vi "test Scheduled Loopback with SDI.vi"(8 "error in":errorcluster, 11 "TestCase in":refnum<class "Single Board Loopback.lvclass">) -> (0 "error out":errorcluster, 3 "TestCase out":refnum<class "Single Board Loopback.lvclass">)   [LabVIEW 2020, in "Single Board Loopback.lvclass"]
uses:
  Single Board Loopback.lvclass
  C:/Users/nitest/Desktop/Git 2020/niveristand-custom-device-testing-tools/VeriStandTestCase/VeriStandTestCase.lvclass
  <vilib>/numeric/Random Number (Range) U64.vi
  <vilib>/numeric/sub_Random U32.vi
  <vilib>/addons/_JKI Toolkits/VI Tester/TestCase.llb/TestCase.lvclass
  niveristand-custom-device-testing-tools/VeriStandTestUtilities/VeriStandTestUtilities.lvlib
  C:/Program Files (x86)/National Instruments/LabVIEW 2020/vi.lib/addons/_JKI Toolkits/VI Tester/TestCase.llb/TestCase.lvclass
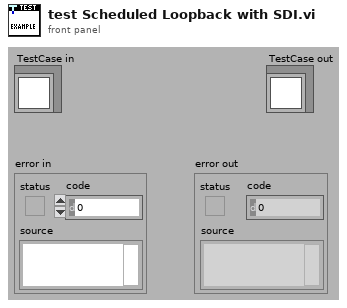
[diagram p1: front panel]
types:
  T1 = typedef "NI_VS Workspace ExecutionAPI.lvlib/WorkspaceAPI.ctl" = refnum<k24>
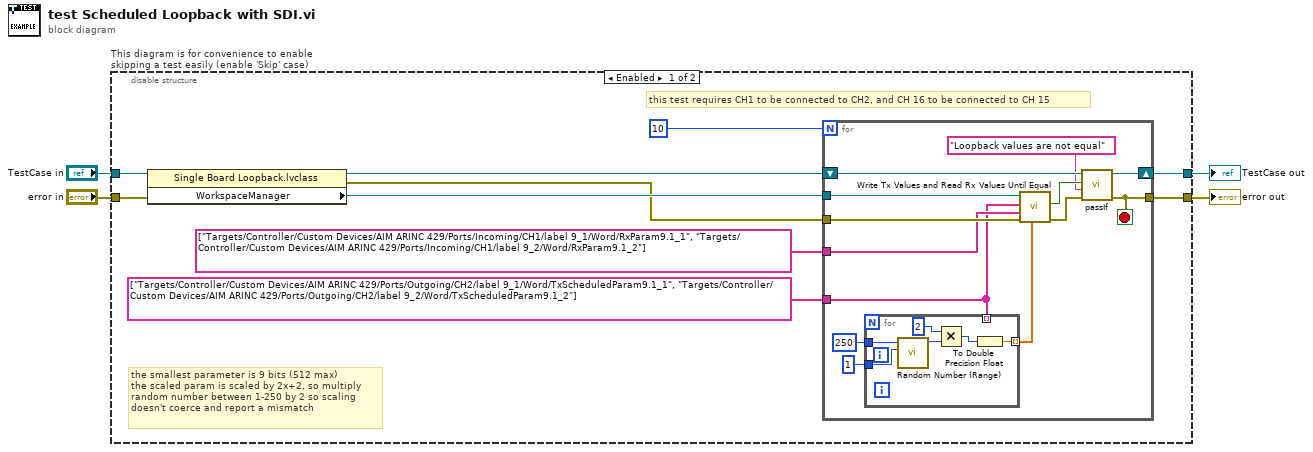
[diagram p0: block diagram]
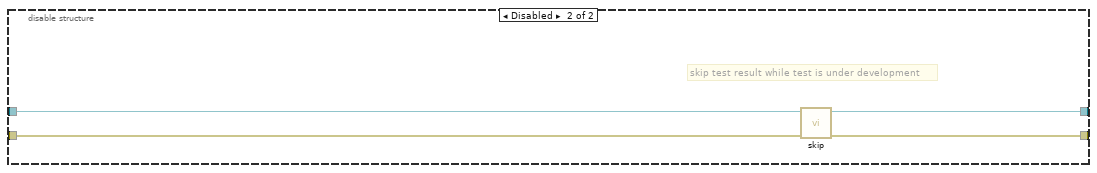
[diagram p2: hidden frame]
diagram:
  n1 = disable-structure "This diagram is for convenience to enable skipping a test easily (enable 'Skip' case)" shown="Enabled" {
    disable-tunnel: "TestCase in" -> [w10 w37]
    disable-tunnel: [w8 w35] -> w1
    disable-tunnel: [w7 w36] -> w3
    disable-tunnel: "error in" -> [w9 w34]
    frame Enabled {
      # "the smallest parameter is 9 bits (512 max)\nthe scaled param is scaled by 2x+2, so multiply \nrandom number between 1-250 by 2 so scaling\ndoesn't coerce and report a mismatch"
      # "this test requires CH1 to be connected to CH2, and CH 16 to be connected to CH 15"
      n2 = property class="Single Board Loopback.lvclass"(reference=w10, error in=w9) -> (reference out=w12:refnum<class "Single Board Loopback.lvclass">, error out=w13:errorcluster, "WorkspaceManager"=w14:T1)
      n3 = for {
        N: 10 -> [_]
        tunnel: string[] ["Targets/Controller/Custom Devices/AIM ARINC 429/Ports/Incoming/CH1/label 9_1/Word/RxParam9.1_1", "Targets/Controller/Custom Devices/AIM ARINC 429/Ports/Incoming/CH1/label 9_2/Word/RxParam9.1_2"] -> [w16]
        tunnel: w14 -> [w27]
        tunnel: w13 -> [w26]
        tunnel: string[] ["Targets/Controller/Custom Devices/AIM ARINC 429/Ports/Outgoing/CH2/label 9_1/Word/TxScheduledParam9.1_1", "Targets/Controller/Custom Devices/AIM ARINC 429/Ports/Outgoing/CH2/label 9_2/Word/TxScheduledParam9.1_2"] -> [w15]
        shift-right: [w23] -> w8
        shift-left: w12 -> [w24]
        tunnel: [w22] -> w7
        stop <- w22 stop-if-true
        n4 = for {
          tunnel: [w32] -> w17 mode=indexing
          tunnel: u64 250 ("upper bound (100)") -> [w31]
          tunnel: u64 1 ("upper bound (100)") -> [w30]
          tunnel: w15 -> [_] mode=indexing
          n5 = call-poly <vilib>:"Random Number (Range).vi"("lower bound (0)"=w30, "upper bound (100)"=w31) -> ("number"=w33:u64)  [unwired: 9 in]
          n6 = Multiply(x=u64 2, y=w33) -> (x*y=w29:u64)
          n7 = To Double Precision Float(number=w29) -> (double precision float=w32:dbl)
        }
        n8 = call "Write Tx Values and Read Rx Values Until Equal.vi"("Tx values"=w17, "error in"=w26, "Rx aliases"=w16, "Tx aliases"=w15, "workspace manager in"=w27) -> ("error out"=w25:errorcluster, "values equal"=w21:bool)  [unwired: 4 in, 1 out]
        n9 = call-dynamic "passIf.vi"("error in (no error)"=w25, "message (\"\")"="Loopback values are not equal" ("message (\"\")"), "pass"=w21, "TestCase in"=w24) -> ("error out"=w22:errorcluster, "TestCase out"=w23:refnum<class "Single Board Loopback.lvclass">)  [unwired: 6 in]
      }
    }
    frame Disabled {
      # "skip test result while test is under development"
      n10 = call <vilib>:"skip.vi"("error in (no error)"=w34, "TestCase in"=w37) -> ("error out"=w36:errorcluster, "TestCase out"=w35:refnum<class "Single Board Loopback.lvclass">)  [unwired: 8 in]
    }
  }
  "error out" <- w3
  "TestCase out" <- w1
